vi "Create All Message Queues.vi"(8 "error in":errorcluster) -> (0 "error out":errorcluster, 3 "Queues":T1)   [LabVIEW 2014, in "Message Queue.lvlib"]
doc: "Creates and initializes message queues"
uses:
  Message Queue.lvlib
  Message Cluster.ctl
  All Message Queues.ctl
  Enqueue Message (Single).vi
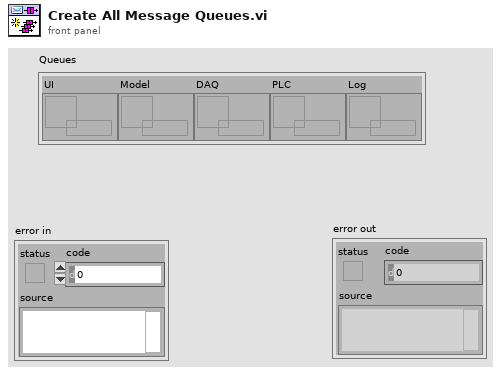
[diagram p1: front panel]
types:
  T1 = typedef "Message Queue.lvlib/All Message Queues.ctl" = cluster{"UI":refnum<queue>, "Model":refnum<queue>, "DAQ":refnum<queue>, "PLC":refnum<queue>, "Log":refnum<queue>}
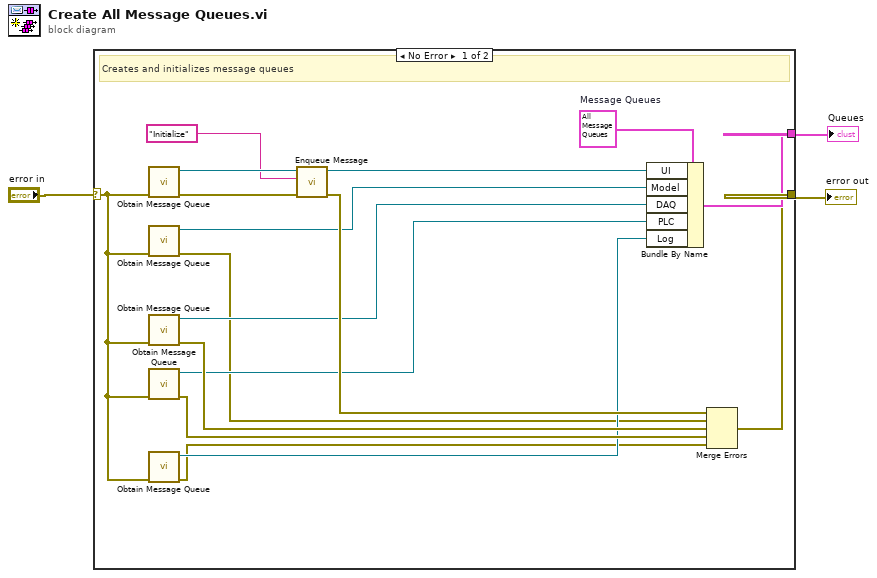
[diagram p0: block diagram]
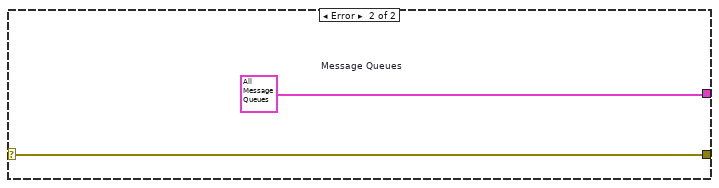
[diagram p2: hidden frame]
diagram:
  n1 = case shown="No Error" "error in" {
    selector: "error in" -> [w13 w22]
    tunnel: [w14 w22] -> w3
    tunnel: [w19 w21] -> w2
    frame No Error {
      w20 = T1 {"UI"=refnum, "Model"=refnum, "DAQ"=refnum, "PLC"=refnum, "Log"=refnum}  # Message Queues
      # "Creates and initializes message queues"
      n2 = call "Obtain Message Queue.vi"("error in (no error)"=w13) -> ("error out"=w18:errorcluster, "Message Queue"=w17:refnum<queue>)  [unwired: 9 in]
      n3 = call "Obtain Message Queue.vi"("error in (no error)"=w13) -> ("error out"=w5:errorcluster, "Message Queue"=w4:refnum<queue>)  [unwired: 9 in]
      n4 = call "Obtain Message Queue.vi"("error in (no error)"=w13) -> ("error out"=w10:errorcluster, "Message Queue"=w11:refnum<queue>)  [unwired: 9 in]
      n5 = call "Obtain Message Queue.vi"("error in (no error)"=w13) -> ("error out"=w8:errorcluster, "Message Queue"=w9:refnum<queue>)  [unwired: 9 in]
      n6 = call "Obtain Message Queue.vi"("error in (no error)"=w13) -> ("error out"=w6:errorcluster, "Message Queue"=w7:refnum<queue>)  [unwired: 9 in]
      n7 = call-poly "Enqueue Message.vi"("error in (no error)"=w18, "Message"="Initialize", "Message Queue"=w17) -> ("error out"=w15:errorcluster, "dup Message Queue"=w16:refnum<queue>)  [unwired: 7 in]
      n8 = Bundle By Name(cluster=w20, "UI"=w16, "Model"=w4, "DAQ"=w11, "PLC"=w9, "Log"=w7) -> (w19:T1)
      n9 = Merge Errors(w15, w5, w10, w8, w6) -> (w14:errorcluster)
    }
    frame Error {
      w21 = T1 {"UI"=refnum, "Model"=refnum, "DAQ"=refnum, "PLC"=refnum, "Log"=refnum}  # Message Queues
    }
  }
  "Queues" <- w2
  "error out" <- w3
